vi "LVClass_DataClient GetImage.vi"(0 "DataClient in":refnum<class "DataClient.lvclass">, 5 "name":string, 7 "Image in":refnum<class "Image.lvclass">, 11 "error in (no error)":errorcluster) -> (4 "DataClient out":refnum<class "DataClient.lvclass">, 8 "Image (dup)":refnum<class "Image.lvclass">, 10 "data_unique_id":i32, 15 "error out":errorcluster)   [LabVIEW 2020, in "DataClient.lvclass"]
doc: "Slopes getter.\n\n--------------------------------------------------------------------------------\n\n<B>clientIn </B> : Client object.\n<B>clientOut </B> : Client object.\n<B>hasoslopes </B> : HasoSlopes object.\n<B>ErrorIn </B> : Error\n<B>ErrorOut </B> : Error\n\n--------------------------------------------------------------------------------"
uses:
  DataClient.lvclass
  Image.lvclass
  DataClient.lvclass/DataClient.ctl
  LVClass_Image Read Image.vi
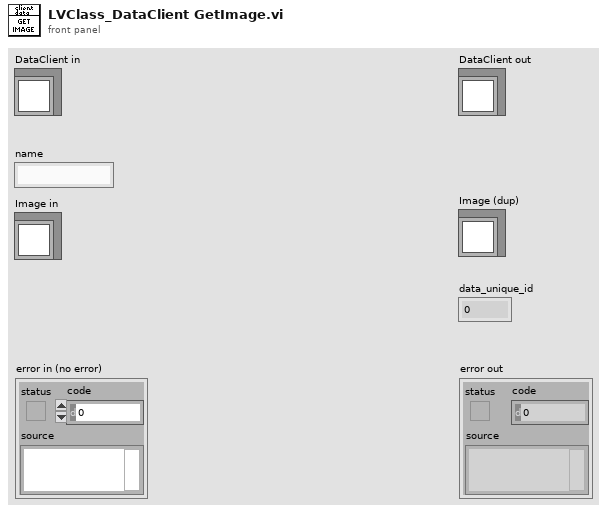
[diagram p1: front panel]
types:
  T1 = typedef "Struct_Image.ctl" = cluster{"Image_Handler":i32, "Number of bits":T2, "ImageSize":T3}
  T2 = typedef "Data alignment enum.ctl" = enum16{"8", "16", "32"}
  T3 = typedef "Point2D.ctl" = cluster{"X":u32, "Y":u32}
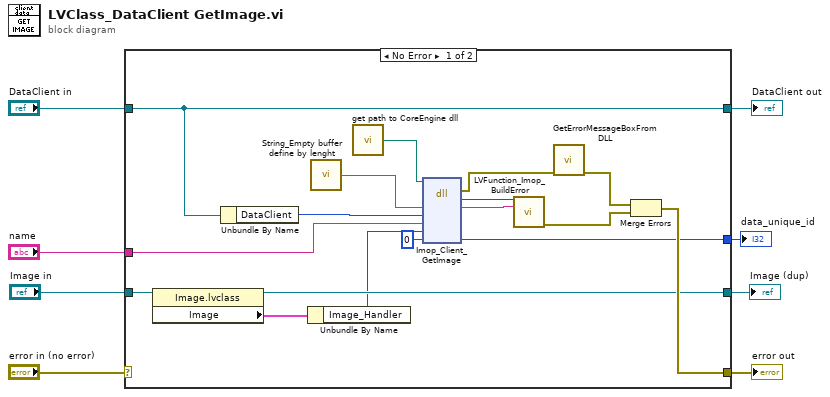
[diagram p0: block diagram]
diagram:
  n1 = case shown="No Error" "error in (no error)" {
    selector: "error in (no error)" -> [_ w28]
    tunnel: [w14 w28] -> w7
    tunnel: [w16 w27] -> w5
    tunnel: "DataClient in" -> [w16 w27]
    tunnel: "Image in" -> [w15 w26]
    tunnel: [w10 w26] -> w3
    tunnel: "name" -> [w13 _]
    tunnel: [w11 _] -> w1
    frame No Error {
      n2 = property class="Image.lvclass"(reference=w15) -> (reference out=w10:refnum<class "Image.lvclass">, "Image"=w25:T1)  [unwired: 1 in, 1 out]
      n3 = Unbundle By Name(w16) -> ("DataClient"=w19:i32)
      n4 = Unbundle By Name(w25) -> ("Image_Handler"=w9:i32)
      n5 = call "String_Empty buffer define by lenght.vi"() -> ("Empty buffer"=w22:string)  [unwired: 1 in]
      n6 = call "get path to CoreEngine dll.vi"() -> ("path to c_interface_vc100.dll"=w21:path)  [unwired: 12 in, 3 out]
      n7 = dll-call lib="D:/soft/HASO_v3/SVN_trunk/ImOpCoreEngine4_LV2011/DLLs/c_interface_vc100.dll" fn="Imop_Client_GetImage"(path in=w21, "message"=w22, "client"=w19, "name"=w13, "Image"=w9, "data_id"=0) -> (error out=w20:errorcluster, "return type"=w24:i32, "message"=w23:string, "data_id"=w11:i32)  [unwired: 5 in, 1 out]
      n8 = call "LVFunction_Imop_BuildError.vi"("code"=w24, "String to Prepend to source (\"\")"=w23) -> ("error out"=w17:errorcluster)  [unwired: 13 in]
      n9 = call "GetErrorMessageBoxFromDLL.vi"("error IN"=w20) -> ("error OUT"=w18:errorcluster)  [unwired: 10 in]
      n10 = Merge Errors(w18, w17) -> (w14:errorcluster)
    }
    frame Error {
    }
  }
  "error out" <- w7
  "DataClient out" <- w5
  "Image (dup)" <- w3
  "data_unique_id" <- w1
